vi "grabAcquire.vi"(0 "HGF_IMAQDevice":refnum<class "HGF_IMAQDevice.lvclass">, 2 "Image In":T1, 3 "Wait for Next Buffer? (Yes)":bool=TRUE, 5 "error in (no error)":errorcluster) -> (14 "dup HGF_IMAQDevice":refnum<class "HGF_IMAQDevice.lvclass">, 16 "Image Out":T1, 17 "Acquired Buffer Number":u32, 19 "error out":errorcluster)   [LabVIEW 2014, in "HGF_IMAQ.lvlib" / "HGF_IMAQDevice.lvclass"]
doc: "Acquires an image from a grab acquisition. Use the grab function for high-speed image acquisition.\n\nWait parameter is ignored by IMAQ for USB."
uses:
  HGF_IMAQDevice.lvclass
  <vilib>/vision/Image Controls.llb/IMAQ Image.ctl
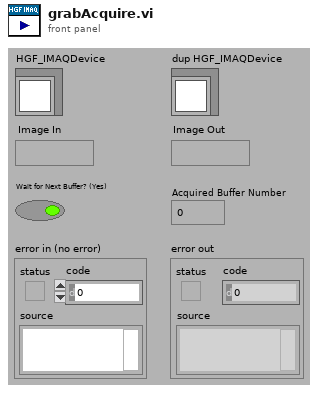
[diagram p1: front panel]
types:
  T1 = typedef "IMAQ Image.ctl" = refnum<image>
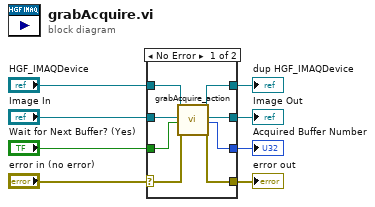
[diagram p0: block diagram]
diagram:
  n1 = case shown="No Error" "error in (no error)" {
    selector: "error in (no error)" -> [w16 w19]
    tunnel: [w15 w19] -> w7
    tunnel: [w11 w18] -> w5
    tunnel: "HGF_IMAQDevice" -> [w12 w18]
    tunnel: [w13 w17] -> w4
    tunnel: "Image In" -> [w14 w17]
    tunnel: "Wait for Next Buffer? (Yes)" -> [w10 _]
    tunnel: [w9 _] -> w1
    frame No Error {
      n2 = call-dynamic "grabAcquire_action.vi"("HGF_IMAQDevice"=w12, "Image In"=w14, "Wait for Next Buffer? (Yes)"=w10, "error in (no error)"=w16) -> ("dup HGF_IMAQDevice"=w11:refnum<class "HGF_IMAQDevice.lvclass">, "Image Out"=w13:T1, "Acquired Buffer Number"=w9:u32, "error out"=w15:errorcluster)  [unwired: 12 out]
    }
    frame Error {
    }
  }
  "error out" <- w7
  "dup HGF_IMAQDevice" <- w5
  "Image Out" <- w4
  "Acquired Buffer Number" <- w1
